vi "e5.4 (hw3).vi"() -> ()   [LabVIEW 2017]
panel:
  in  "STOP Button":bool
  out "Loop Iteration":dbl
  in  "Input (N)":dbl=1.0 min=1.0
  # "Problem E 5.4 (HW 3)"
  # "Input N has to be greater than 0"
  # "Patrik Sokolowski"
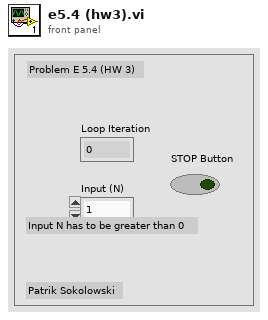
[diagram p1: front panel]
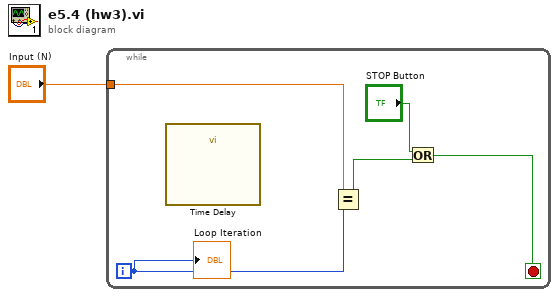
[diagram p0: block diagram]
diagram:
  n1 = while {
    tunnel: "Input (N)" -> [w3]
    i -> [w6]
    stop <- w4 stop-if-true
    n2 = call "Time Delay"() -> ()  [unwired: 11 in, 1 out]
    n3 = Equal?(x=w3, y=w6) -> (x = y?=w5:bool)
    n4 = Or(x="STOP Button", y=w5) -> (x .or. y?=w4:bool)
    "Loop Iteration" <- w6
  }
